vi "AVTCP-Start Recording.vi"(11 "filepath":string) -> ()   [LabVIEW 2020]
uses:
  Sub VIs/AVTCP-FGV Action.ctl
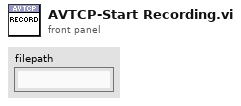
[diagram p1: front panel]
types:
  T1 = typedef "AVTCP-FGV Action.ctl" = enum16{"Init", "Write", "Read"}
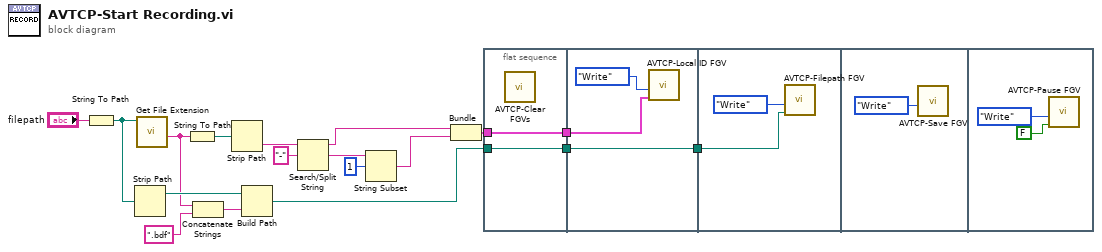
[diagram p0: block diagram]
diagram:
  n1 = String To Path(string="filepath") -> (path=w11:path)
  n2 = Strip Path(path=w11) -> (stripped path=w14:path)  [unwired: 1 out]
  n3 = call <vilib>:"Get File Extension.vi"("file"=w11) -> ("filename without extension"=w13:string)  [unwired: 6 in, 4 out]
  n4 = String To Path(string=w13) -> (path=w15:path)
  n5 = Concatenate Strings(w13, ".bdf") -> (w7:string)
  n6 = Strip Path(path=w15) -> (name=w18:string)  [unwired: 1 out]
  n7 = Build Path(base path=w14, name or relative path=w7) -> (appended path=w1:path)
  n8 = Search/Split String(string=w18, search string/char (-)="-") -> (substring before match=w10:string, match + rest of string=w9:string)  [unwired: 1 in, 1 out]
  n9 = String Subset(string=w9, offset (0)=1) -> (substring=w8:string)  [unwired: 1 in]
  n10 = Bundle("name"=w10, "name"=w8) -> (w5:cluster{"name":string, "name":string})  [unwired: 1 in]
  n11 = flat-sequence {
    tunnel: w5 -> [w20]
    tunnel: [w20] -> w4
    tunnel: [w19] -> w2
    tunnel: w1 -> [w19]
    tunnel: w4 -> [w22]
    tunnel: [w21] -> w3
    tunnel: w2 -> [w21]
    tunnel: w3 -> [w24]
    frame #0 {
      n12 = call "AVTCP-Clear FGVs.vi"() -> ()  [unwired: 12 in]
    }
    frame #1 {
      n13 = call "AVTCP-Local ID FGV.vi"("Value in"=w22, "Action"=AVTCP-FGV_Action."Write") -> ()  [unwired: 4 in, 2 out]
    }
    frame #2 {
      n14 = call "AVTCP-Filepath FGV.vi"("Value in"=w24, "Action"=AVTCP-FGV_Action."Write") -> ()  [unwired: 5 in, 1 out]
    }
    frame #3 {
      n15 = call "AVTCP-Save FGV.vi"("Action"=AVTCP-FGV_Action."Write") -> ()  [unwired: 6 in, 1 out]
    }
    frame #4 {
      n16 = call "AVTCP-Pause FGV.vi"("Value in"=FALSE, "Action"=AVTCP-FGV_Action."Write") -> ()  [unwired: 5 in, 1 out]
    }
  }
